vi "Process Image for Target.vi"(0 "Src Image":T2, 1 "Color Mode":u16(ring)=2 items=["RGB", "HSL", "HSV", "HSI"], 9 "Color Components":T3={"Hue"={110.0, 142.0}, "Sat"={138.0, 255.0}, "Val"={139.0, 198.0}} {"Val" scale=0.0..255.0; "Sat" scale=0.0..255.0; "Hue" scale=0.0..255.0 scale format="%#_3g"}, 11 "Area Cutoff %":dbl=0.05) -> (4 "Src Image Out":T2, 8 "Threshold":T2, 15 "Particles":T1(array[cluster]))   [LabVIEW 2013]
doc: "Use color, rectangularity, and aspect ratio to identify and describe potential strips of retroreflective material within the image."
uses:
  <vilib>/vision/Image Controls.llb/IMAQ Image.ctl
  <vilib>/vision/NI_Vision_Development_Module.lvlib
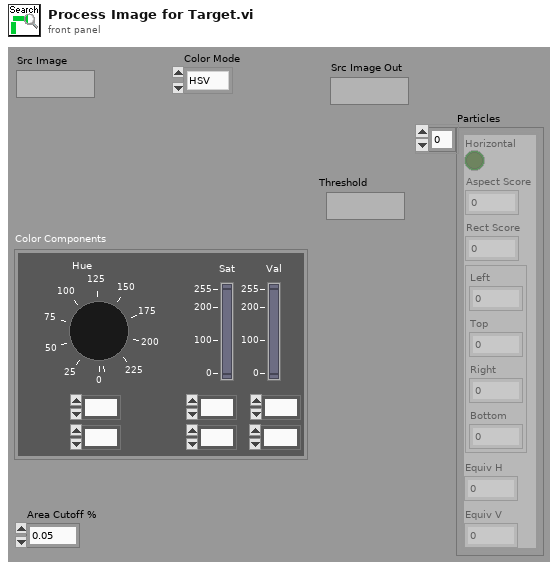
[diagram p1: front panel]
types:
  T1 = cluster{"Horizontal":bool, "Aspect Score":dbl, "Rect Score":dbl, cluster{"Left":dbl, "Top":dbl, "Right":dbl, "Bottom":dbl}, "Equiv H":dbl, "Equiv V":dbl}[]
  T2 = typedef "IMAQ Image.ctl" = refnum<image>
  T3 = cluster{"Hue":cluster{dbl, dbl}, "Sat":cluster{dbl, dbl}, "Val":cluster{dbl, dbl}}
  T4 = typedef "Particle Parameters" = i32
  T5 = typedef "Image Type" = u32
  T6 = cluster{"Numeric":dbl, "Numeric":dbl, "Numeric":dbl, "Numeric":dbl}
  T7 = cluster{"Horizontal":bool, "Score":dbl, "Score":dbl, cluster{"Numeric":dbl, "Numeric":dbl, "Numeric":dbl, "Numeric":dbl}, "Numeric":dbl, "Numeric":dbl}
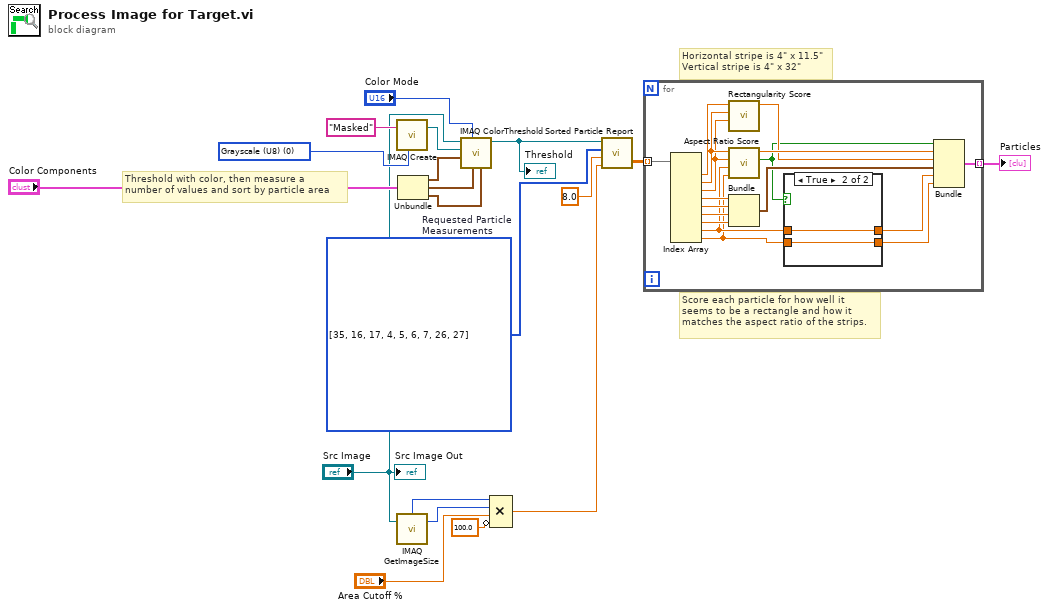
[diagram p0: block diagram]
diagram:
  w8 = T4[] [35, 16, 17, 4, 5, 6, 7, 26, 27] items=["Center of Mass X", "Center of Mass Y", "First Pixel X", "First Pixel Y", "Bounding Rect Left", "Bounding Rect Top", "Bounding Rect Right", "Bounding Rect Bottom", "Max Feret Diameter Start X", "Max Feret Diameter Start Y", "Max Feret Diameter End X", "Max Feret Diameter End Y", "Max Horiz. Segment Length Left", "Max Horiz. Segment Length Right", "Max Horiz. Segment Length Row", "-", "Bounding Rect Width", "Bounding Rect Height", "Bounding Rect Diagonal", "Perimeter", "Convex Hull Perimeter", "Holes' Perimeter", "Max Feret Diameter", "Equivalent Ellipse Major Axis", "Equivalent Ellipse Minor Axis", "Equivalent Ellipse Minor Axis (Feret)", "Equivalent Rect Long Side", "Equivalent Rect Short Side", "Equivalent Rect Diagonal", "Equivalent Rect Short Side (Feret)", "Average Horiz. Segment Length", "Average Vert. Segment Length", "Hydraulic Radius", "Waddel Disk Diameter", "-", "Area", "Holes' Area", "Particle & Holes' Area", "Convex Hull Area", "Image Area", "-", "Number of Holes", "Number of Horiz. Segments", "Number of Vert. Segments", "-", "Orientation", "Max Feret Diameter Orientation", "-", "% Area/Image Area", "% Area/(Particle & Holes' Area)", "Ratio of Equivalent Ellipse Axes", "Ratio of Equivalent Rect Sides", "-", "Elongation Factor", "Compactness Factor", "Heywood Circularity Factor", "Type Factor", "-", "Sum X", "Sum Y", "Sum XX", "Sum XY", "Sum YY", "Sum XXX", "Sum XXY", "Sum XYY", "Sum YYY", "-", "Moment of Inertia XX", "Moment of Inertia XY", "Moment of Inertia YY", "Moment of Inertia XXX", "Moment of Inertia XXY", "Moment of Inertia XYY", "Moment of Inertia YYY", "Norm. Moment of Inertia XX", "Norm. Moment of Inertia XY", "Norm. Moment of Inertia YY", "Norm. Moment of Inertia XXX", "Norm. Moment of Inertia XXY", "Norm. Moment of Inertia XYY", "Norm. Moment of Inertia YYY", "Hu Moment 1", "Hu Moment 2", "Hu Moment 3", "Hu Moment 4", "Hu Moment 5", "Hu Moment 6", "Hu Moment 7"]  # Requested Particle Measurements
  w17 = T5 0 items=["Grayscale (U8)", "Grayscale (I16)", "Grayscale (SGL)", "Complex (CSG)", "RGB (U32)", "HSL (U32)", "RGB (U64)", "Grayscale (U16)"] ("Image Type")
  # "Score each particle for how well it\nseems to be a rectangle and how it\nmatches the aspect ratio of the strips."
  # "Horizontal stripe is 4\" x 11.5\"\nVertical stripe is 4\" x 32\""
  # "Threshold with color, then measure a\nnumber of values and sort by particle area"
  n1 = call "IMAQ Create"("Image Name"="Masked", "Image Type"=w17) -> ("New Image"=w15:T2)  [unwired: 3 in, 1 out]
  n2 = call "IMAQ GetImageSize"("Image"="Src Image") -> ("Y Resolution"=w12:i32, "X Resolution"=w13:i32)  [unwired: 3 in, 1 out]
  n3 = Unbundle("Color Components") -> ("Hue"=w1:cluster{dbl, dbl}, "Sat"=w2:cluster{dbl, dbl}, "Val"=w3:cluster{dbl, dbl})
  n4 = call "IMAQ ColorThreshold"("Blue or Luma or Val or Inten Range"=w3, "Green or Sat Range"=w2, "Color Mode"="Color Mode", "Red or Hue Range"=w1, "Image Dst"=w15, "Image Src"="Src Image") -> ("Image Dst Out"=w5:T2)  [unwired: 4 in, 1 out]
  "Threshold" <- w5
  n5 = Compound Arithmetic op=MULTIPLY(w13, w12, "Area Cutoff %", invert 100.0 ("value")) -> (w10:dbl)
  n6 = call "Sorted Particle Report.vi"("Area Size Limit"=w10, "Particle Count Limit"=8.0, "Pixel Measurements"=w8, "Image in"=w5) -> ("Sorted Data"=w7:dbl[][])  [unwired: 1 out]
  n7 = for {
    tunnel: w7 -> [w36] mode=indexing
    tunnel: [w26] -> w4 mode=indexing
    n8 = Index Array(array=w36) -> (element #1=w35:dbl, element #2=w30:dbl, element #3=w29:dbl, element #4=w34:dbl, element #5=w33:dbl, element #6=w32:dbl, element #7=w31:dbl, element #8=w21:dbl, element #9=w20:dbl)  [unwired: 9 in]
    n9 = call "Rectangularity Score.vi"("Height"=w29, "Width"=w30, "Area"=w35) -> ("Score"=w27:dbl)  [unwired: 8 in]
    n10 = call "Aspect Ratio Score.vi"("Equivalent Rect Short"=w20, "Equivalent Rect Long"=w21, "Height"=w29, "Width"=w30) -> ("Horizontal"=w22:bool, "Score"=w28:dbl)  [unwired: 6 in]
    n11 = Bundle("Numeric"=w34, "Numeric"=w33, "Numeric"=w32, "Numeric"=w31) -> (w25:T6)  [unwired: 1 out]
    n12 = case shown="True" w22 {
      tunnel: w20 -> [w37 w40]
      tunnel: w21 -> [w38 w39]
      tunnel: [w38 w40] -> w24
      tunnel: [w37 w39] -> w23
      frame False {
      }
      frame True {
      }
    }
    n13 = Bundle("Horizontal"=w22, "Score"=w28, "Score"=w27, w25, "Numeric"=w23, "Numeric"=w24) -> (w26:T7)  [unwired: 1 out]
  }
  "Particles" <- w4
  "Src Image Out" <- "Src Image"
